vi "BRig_dataLC_Cue2_First_OnOff_l1.vi"() -> (2 "output_Cue2_First_OnOff":i32)   [LabVIEW 2014]
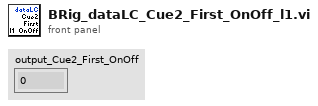
[diagram p1: front panel]
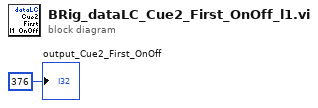
[diagram p0: block diagram]
diagram:
  "output_Cue2_First_OnOff" <- 376 ("output_iBlock")
